vi "Get Parameter Value by Name (U32).vi"(8 "Default Value":u32, 9 "Parameter":string, 10 "Parameter Array in":string[](array[string])) -> (1 "Value":u32, 2 "Found?":bool, 3 "Parameter Array Out":string[](array[string]))   [LabVIEW 2014]
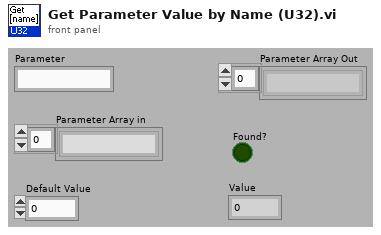
[diagram p1: front panel]
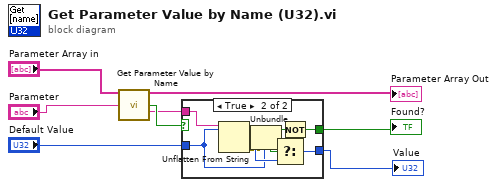
[diagram p0: block diagram]
diagram:
  n1 = call "Get Parameter Value by Name.vi"("Parameter Array"="Parameter Array in", "Parameter Name"="Parameter") -> ("Parameter Array Out"=→"Parameter Array Out":string[], "Found?"=w5:bool, "Flattened Value"=w4:string)  [unwired: 11 in]
  n2 = case shown="True" w5 {
    selector: w5 -> [w9 _]
    tunnel: w4 -> [_ w17]
    tunnel: "Default Value" -> [w10 w14]
    tunnel: [w10 w15] -> w8
    tunnel: [w9 w12] -> w1
    frame False {
    }
    frame True {
      n3 = Unflatten From String(type=w14, binary string=w17) -> (value=w16:u32, error out=w11:errorcluster)  [unwired: 3 in, 1 out]
      n4 = Unbundle(w11) -> ("status"=w13:bool)  [unwired: 2 out]
      n5 = Select(t=w14, s=w13, f=w16) -> (s? t:f=w15:u32)
      n6 = Not(x=w13) -> (.not. x?=w12:bool)
    }
  }
  "Value" <- w8
  "Found?" <- w1
